vi "Auto 6.vi"(8 "Error In":errorcluster) -> (0 "Error Out":errorcluster)   [LabVIEW 2014]
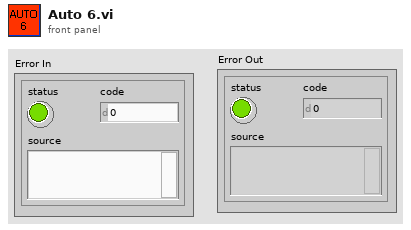
[diagram p1: front panel]
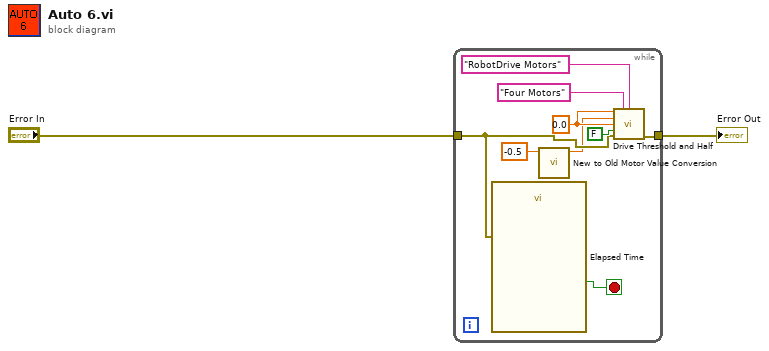
[diagram p0: block diagram]
diagram:
  n1 = while {
    tunnel: "Error In" -> [w5]
    tunnel: [w8] -> w2
    stop <- w6 stop-if-true
    w7 = 0.0 ("Arm Value")
    n2 = call "Elapsed Time"("error in (no error)"=w5) -> ("Time has Elapsed"=w6:bool)  [unwired: 11 in, 7 out]
    n3 = call "New to Old Motor Value Conversion.vi"("Motor Value In"=-0.5 ("X In")) -> ("New to Old Conversion Value Out"=w3:dbl)  [unwired: 9 in, 1 out]
    n4 = call "Drive Threshold and Half.vi"("X In"=w7, "Drive refnum name"="Four Motors" ("refnum name"), "Send to DB Name"="RobotDrive Motors" ("Name"), "Y In"=w3, "R In"=w7, "Speed Toggle"=FALSE ("Grabber Open/Close"), "Error In"=w5) -> ("Error Out"=w8:errorcluster)  [unwired: 8 in]
  }
  "Error Out" <- w2
